vi "Configure Trigger (Logic & Digital Channel).vi"(0 "VISA resource name":refnum<visa-resource-name>, 1 "Minimum Time (2E-9 s)":dbl=2e-09, 5 "Digital Channel (0: Digital Channel 0)":i32(ring) items=["Digital Channel 0", "Digital Channel 1", "Digital Channel 2", "Digital Channel 3", "Digital Channel 4", "Digital Channel 5", "Digital Channel 6", "Digital Channel 7", "Digital Channel 8", "Digital Channel 9", "Digital Channel 10", "Digital Channel 11", "Digital Channel 12", "Digital Channel 13", "Digital Channel 14", "Digital Channel 15"], 7 "Logic Pattern Input (2: Do Not Care)":i32(ring)=2 items=["Logic High", "Logic Low", "Do Not Care"], 9 "Logic Trigger Threshold (1.4 V)":dbl=1.4, 11 "error in (no error)":errorcluster, 12 "Maximum Time (8E-9 s)":dbl=8e-09) -> (4 "VISA resource name out":refnum<visa-resource-name>, 15 "error out":errorcluster)   [LabVIEW 2017, in "Scope.lvlib" / "Tektronix DPO MSO 2000 4000 Series.lvlib"]
doc: "Configures logic trigger settings for digital channel of an oscilloscope.\n\n<B>Note:</B>\n\nThis VI is only applicable to <B>MDO series</B> oscilloscopes."
uses:
  Tektronix DPO MSO 2000 4000 Series.lvlib
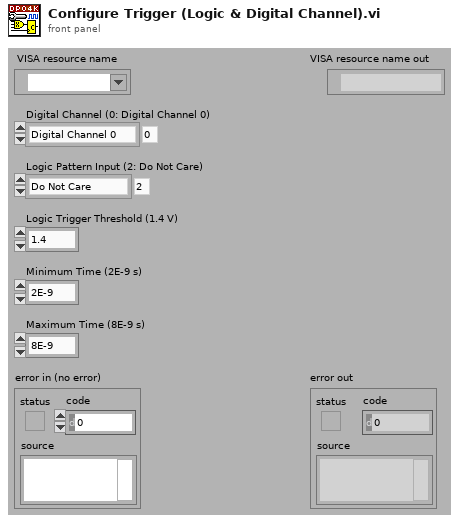
[diagram p1: front panel]
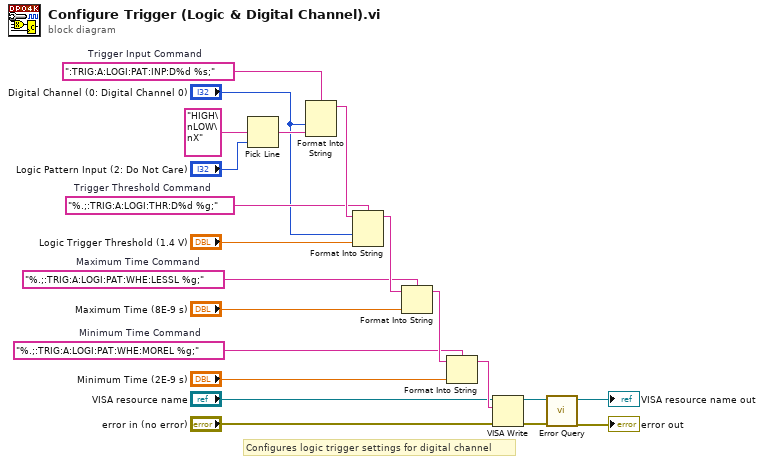
[diagram p0: block diagram]
diagram:
  w10 = "%.;:TRIG:A:LOGI:PAT:WHE:MOREL %g;"  # Minimum Time Command
  w13 = "%.;:TRIG:A:LOGI:PAT:WHE:LESSL %g;"  # Maximum Time Command
  w16 = "%.;:TRIG:A:LOGI:THR:D%d %g;"  # Trigger Threshold Command
  w19 = ":TRIG:A:LOGI:PAT:INP:D%d %s;"  # Trigger Input Command
  # "Configures logic trigger settings for digital channel"
  n1 = Pick Line(multi-line string="HIGH\nLOW\nX", line index="Logic Pattern Input (2: Do Not Care)") -> (output string=w18:string)  [unwired: 1 in]
  n2 = Format Into String(format string=w19, "Digital Channel (0: Digital Channel 0)", w18) -> (resulting string=w17:string)  [unwired: 2 in, 1 out]
  n3 = Format Into String(format string=w16, initial string=w17, "Digital Channel (0: Digital Channel 0)", "Logic Trigger Threshold (1.4 V)") -> (resulting string=w14:string)  [unwired: 1 in, 1 out]
  n4 = Format Into String(format string=w13, initial string=w14, "Maximum Time (8E-9 s)") -> (resulting string=w11:string)  [unwired: 1 in, 1 out]
  n5 = Format Into String(format string=w10, initial string=w11, "Minimum Time (2E-9 s)") -> (resulting string=w8:string)  [unwired: 1 in, 1 out]
  n6 = VISA Write(VISA resource name="VISA resource name", write buffer=w8, error in (no error)="error in (no error)") -> (VISA resource name out=w5:refnum<visa-resource-name>, error out=w4:errorcluster)  [unwired: 1 out]
  n7 = call "Error Query.vi"("error in (no error)"=w4, "VISA resource name"=w5) -> ("error out"=→"error out":errorcluster, "VISA resource name out"=→"VISA resource name out":refnum<visa-resource-name>)  [unwired: 6 in, 2 out]
